vi "Create Map Attributes.vi"(11 "Path":path) -> (3 "Root Attributes":map{string, string}(c390))   [LabVIEW 2019, in "Panther Dashboard.lvlib"]
uses:
  Panther Dashboard.lvlib
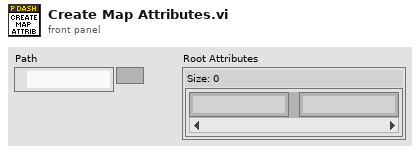
[diagram p1: front panel]
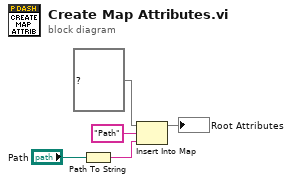
[diagram p0: block diagram]
diagram:
  n1 = Path To String(path="Path") -> (string=w4:string)
  n2 = Insert Into Map(map in=map{string, string} {} ("Root Attributes"), key="Path", value=w4) -> (map out=→"Root Attributes":map{string, string})  [unwired: 2 out]
